vi "readout test plot.vi"() -> ()   [LabVIEW 2021]
panel:
  out "error out":errorcluster
  in  "Stop":bool
  out "IQ vs time":dbl[][](graph)
  out "Mag vs index":dbl[](graph)
  out "Q":T1(graph)
  out "I":T1(graph)
  out "Phase":T1(graph)
  out "Mag":T1(graph)
  in  "error in (no error)":errorcluster
  in  "path":path=path "C:/Users/yg/Desktop/tmp/20230322-230510 test_readout.h5"
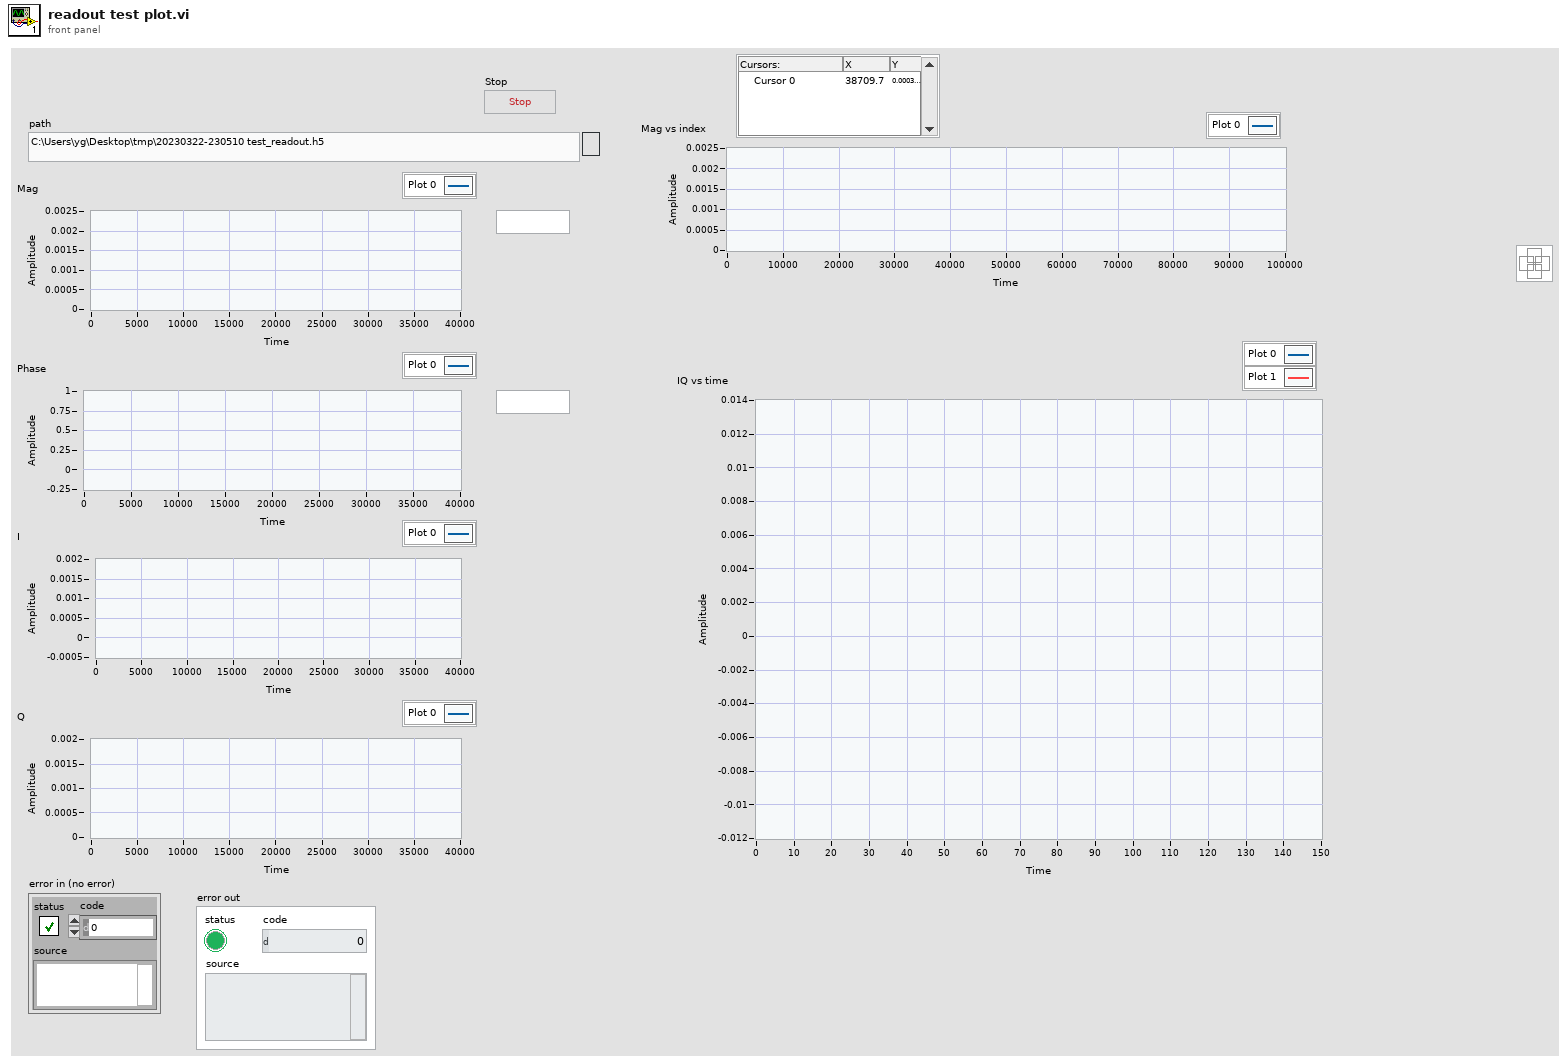
[diagram p1: front panel]
types:
  T1 = cluster{" Integral out":dbl[], " Integral out":dbl[]}
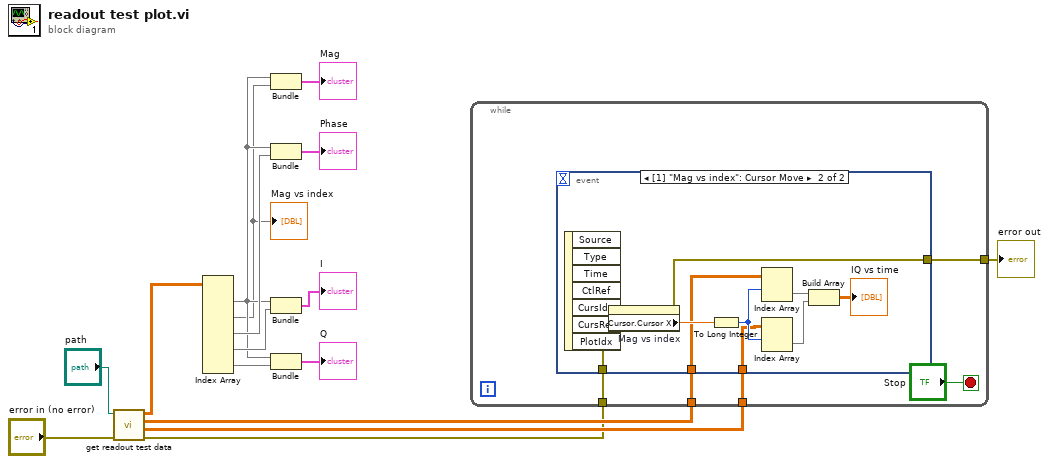
[diagram p0: block diagram]
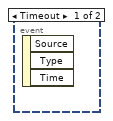
[diagram p2: hidden frame]
diagram:
  n1 = call "get readout test data.vi"("error in (no error)"="error in (no error)", "path"="path") -> ("error out"=w2:errorcluster, "q wave"=w4:dbl[][], "i wave"=w3:dbl[][], "Integral out"=w14:dbl[][])  [unwired: 6 in]
  n2 = Index Array(array=w14) -> (element #1=w8:dbl[], element #2=w5:dbl[], element #3=w12:dbl[], element #4=w10:dbl[], element #5=w7:dbl[])  [unwired: 10 in]
  "Mag vs index" <- w5
  n3 = Bundle("Integral out"=w8, "Integral out"=w5) -> (→"Mag":T1)  [unwired: 1 in]
  n4 = Bundle("Integral out"=w8, "Integral out"=w12) -> (→"Phase":T1)  [unwired: 1 in]
  n5 = Bundle("Integral out"=w8, "Integral out"=w10) -> (→"I":T1)  [unwired: 1 in]
  n6 = Bundle("Integral out"=w8, "Integral out"=w7) -> (→"Q":T1)  [unwired: 1 in]
  n7 = while {
    tunnel: w4 -> [w21]
    tunnel: w3 -> [w20]
    tunnel: w2 -> [w19]
    tunnel: [w17] -> w1
    stop <- "Stop" stop-if-true
    n8 = event shown="[1] \"Mag vs index\": Cursor Move" {
      selector: _ -> [_ _]
      dyn-events: _ -> [_ _]
      timeout: _ -> [_ _]
      tunnel: w21 -> [_ w25]
      tunnel: w20 -> [_ w24]
      tunnel: w19 -> [_ w23]
      tunnel: [_ w22] -> w17
      event Timeout {
        n9 = event-data() -> ()  [unwired: 1 in, 3 out]
      }
      event "Mag vs index": Cursor Move {
        n10 = event-data() -> ()  [unwired: 1 in, 7 out]
        n11 = property on="Mag vs index" class="WFGraph (strict)"(error in=w23) -> (error out=w22:errorcluster, "Cursor.Cursor X"=w26:dbl)  [unwired: 1 in, 1 out]
        n12 = To Long Integer(number=w26) -> (32bit integer=w27:i32)
        n13 = Index Array(array=w24, index (row)=w27) -> (element=w28:dbl[])  [unwired: 1 in]
        n14 = Index Array(array=w25, index (row)=w27) -> (element=w29:dbl[])  [unwired: 1 in]
        n15 = Build Array(w28, w29) -> (→"IQ vs time":dbl[][])
      }
    }
  }
  "error out" <- w1
